vi "Set Proportional Gain.vi"(4 "error in (no error)":errorcluster, 5 "Kp (0)":dbl min=0.0 max=2000000000.0 format="%.6g", 6 "Axis (1)":i32=1 min=1 max=3, 7 "VISA resource name":refnum<visa-resource-name>) -> (0 "error out":errorcluster, 3 "VISA resource name out":refnum<visa-resource-name>)   [LabVIEW 2014, in "Newport ESP301.lvlib"]
doc: "This command sets the proportional gain factor Kp of the PID closed loop. It is\nactive for any DC servo based motion device that has been selected to operate in closed loop.\nThe command can be sent at any time but it has no effect until the UF (updatefilter)is received.\nSee the \"Servo Tuning\" chapter (ESP301 User's manual.pdf) on how to adjust the PID filter parameters."
uses:
  Newport ESP301.lvlib
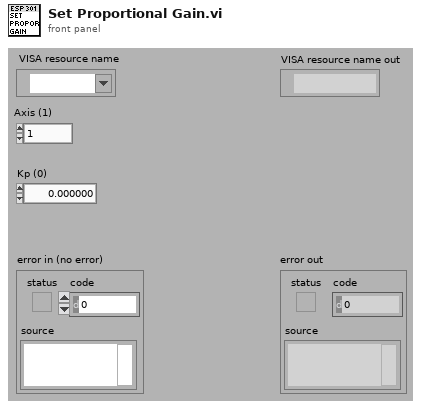
[diagram p1: front panel]
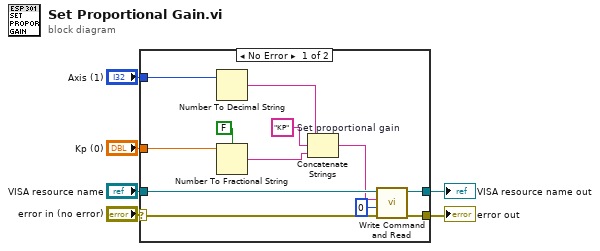
[diagram p0: block diagram]
diagram:
  n1 = case shown="No Error" "error in (no error)" {
    selector: "error in (no error)" -> [w15 w20]
    tunnel: [w17 w20] -> w6
    tunnel: "VISA resource name" -> [w18 w19]
    tunnel: [w16 w19] -> w5
    tunnel: "Kp (0)" -> [w14 _]
    tunnel: "Axis (1)" -> [w13 _]
    frame No Error {
      w12 = "KP"  # Set proportional gain
      n2 = Number To Decimal String(number=w13) -> (decimal integer string=w11:string)  [unwired: 1 in]
      n3 = Number To Fractional String(use system decimal point (T)=FALSE ("utiliser le séparateur décimal du système (V)"), number=w14) -> (F-format string=w10:string)  [unwired: 2 in]
      n4 = Concatenate Strings(w11, w12, w10) -> (w9:string)
      n5 = call "Write Command and Read.vi"("error in (no error)"=w15, "Bytes to read (100)"=u32 0, "Command"=w9, "VISA resource name"=w18) -> ("error out"=w17:errorcluster, "VISA resource name out"=w16:refnum<visa-resource-name>)  [unwired: 3 in, 1 out]
    }
    frame Error {
    }
  }
  "error out" <- w6
  "VISA resource name out" <- w5
